vi "TCP IP Parse CutPower.vi"(11 "JSON in":string) -> (2 "Cut Power":string, 3 "JSON out":string)   [LabVIEW 2015]
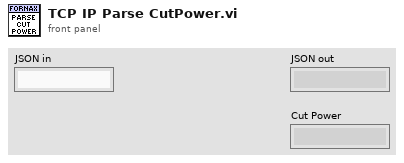
[diagram p1: front panel]
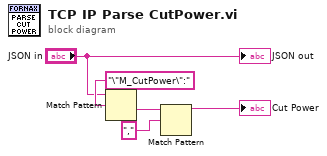
[diagram p0: block diagram]
diagram:
  n1 = Match Pattern(string="JSON in", regular expression="\"M_CutPower\":") -> (after substring=w3:string)  [unwired: 1 in, 3 out]
  n2 = Match Pattern(string=w3, regular expression=",") -> (before substring=→"Cut Power":string)  [unwired: 1 in, 3 out]
  "JSON out" <- "JSON in"
